vi "Session_from_previous_session_dialog.vi"(8 "Current Session Information":T4={"CollectionOfPoints"=[], "Instrument"=enum."Unknown", "CollectionFile"=path "kfaj;ldkfja;f", "Session Name/ID"="", "SessionNotes"=""}) -> (0 "Current Session Information Out":T4={"CollectionOfPoints"=[], "Instrument"=enum."Unknown", "CollectionFile"=path "kfaj;ldkfja;f", "Session Name/ID"="", "SessionNotes"=""}, 3 "Cancelled?":bool)   [LabVIEW 2011]
doc: "Use this template to create a dialog box. This template polls the state of the buttons on the front panel and does not use events. Use the Dialog Using Events template (not available in the Base package) to create a dialog box with event handling."
uses:
  cm2nm_sample_set.ctl
  cm2nm_coordinate_information_v2.ctl
  Instrument_type_enum_v2.ctl
  <vilib>/Analysis/Matrix/Datatypes/RealMatrix.ctl
  <vilib>/Analysis/Matrix/NI_Matrix.lvlib
panel:
  out "transformed with error":T1[](array[typedef])
  in  "Induce_error":dbl
  out "transformed":T1[](array[typedef])
  out "String":string
  out "B - vector offset":T2=[[-50940.89375198816], [16651.91756507725], [483.99442685727536]]
  out "A - Transformation Matrix":T2=[[774.391778229561, 631.2948989068436, 0.0], [-630.6602275509395, 772.5947325435925, 0.0], [2.0151348362659673, -7.982499934864615, 0.0]]
  out "Chosen Array":T1[](array[typedef])
  in  "Azimuth(deg)":dbl
  in  "Elevation (deg)":dbl
  in  "Scale":dbl
  in  "Z-off":dbl
  in  "Y-off":dbl
  in  "X-off":dbl
  in  "ChooseSpots":T3(array[cluster])
  in  "Cancel":bool
  in  "OK":bool
  # "Add the contents of your dialog here.\n\nTip: use controls from the System category of the Controls \npalette for professional appearance.\n\nReplace this text with your own, or delete this label."
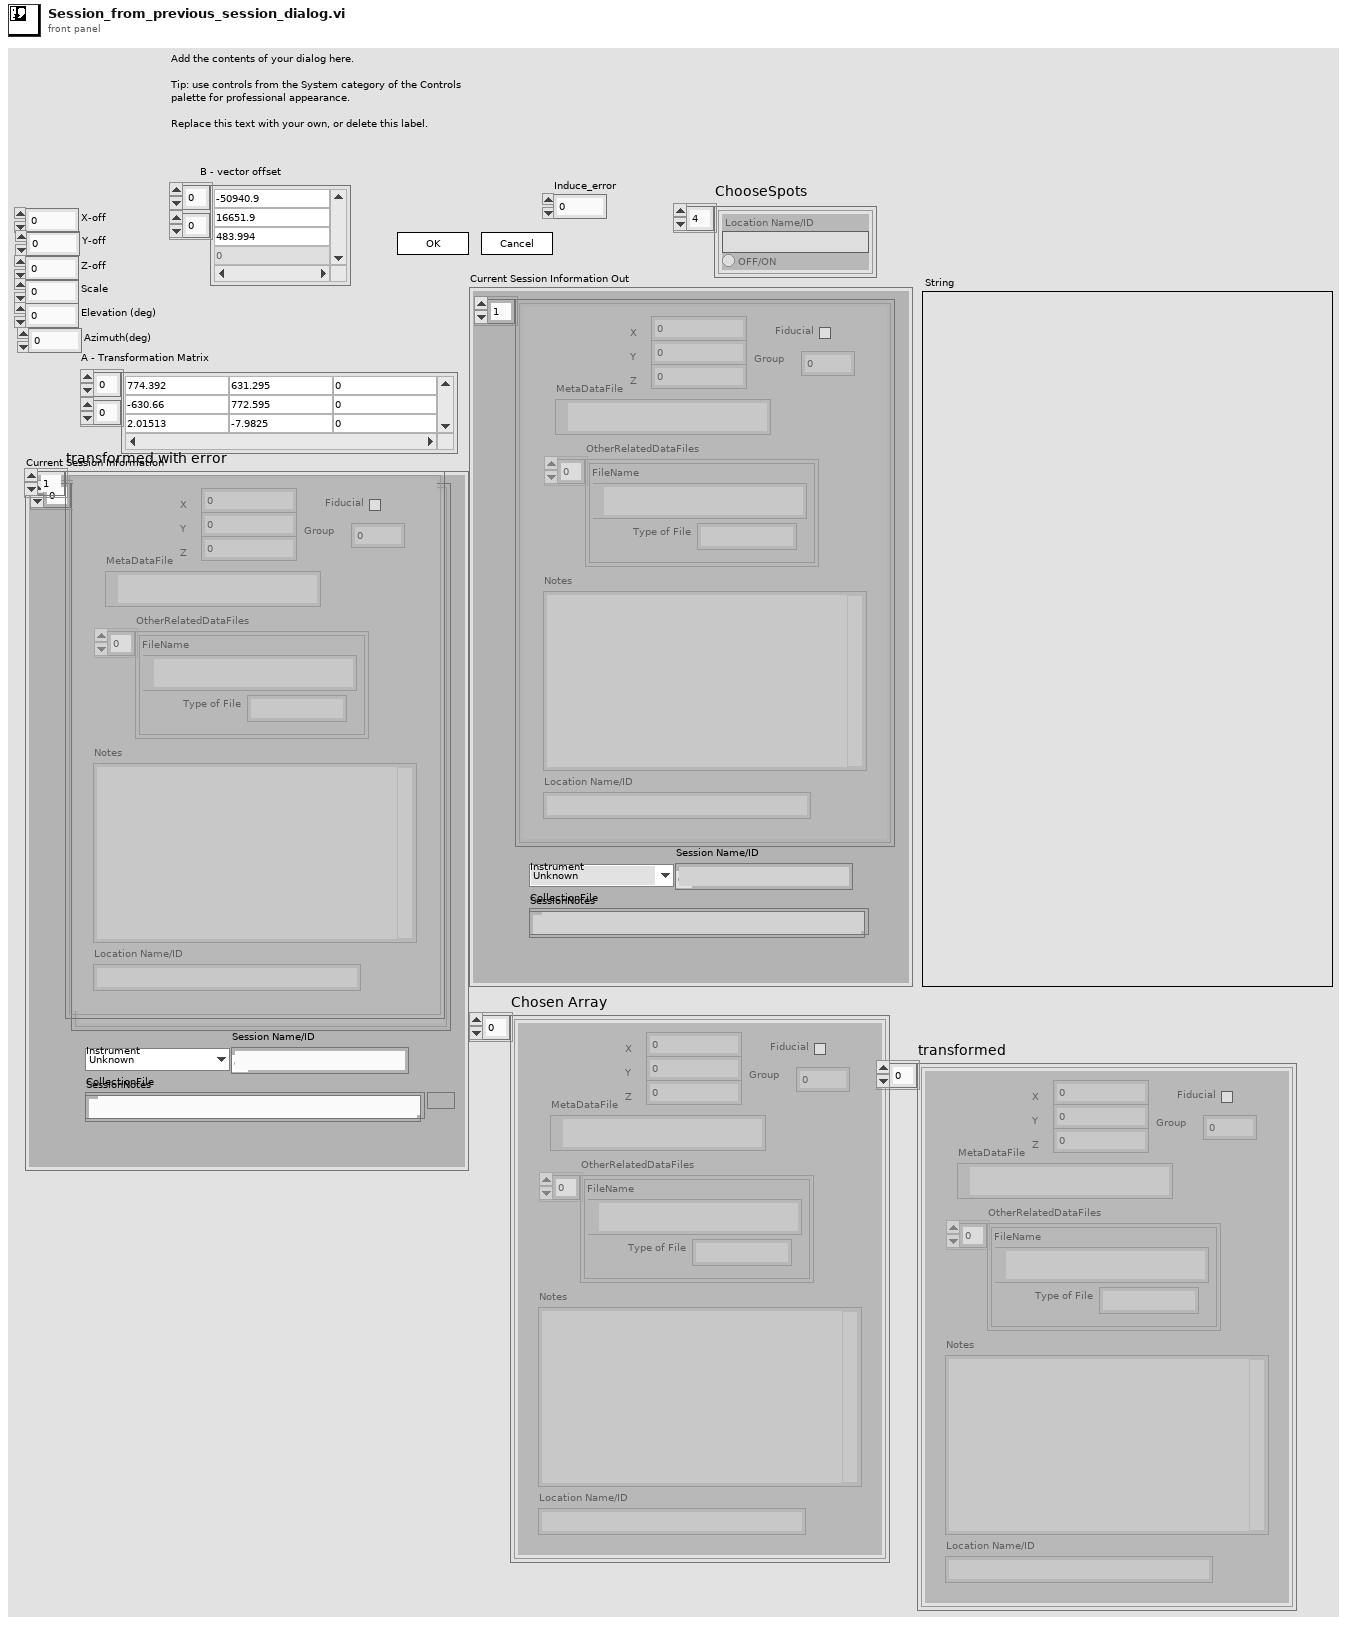
[diagram p1: front panel]
types:
  T1 = typedef "cm2nm_coordinate_information_v2.ctl" = cluster{"MetaDataFile":path, "X":dbl, "Y":dbl, "Z":dbl, "Group":i32, "Rotation":dbl[unit], "Fiducial":bool, "Magnification":dbl, "Working_Distance":dbl, "Notes":string, "Location Name/ID":string, "OtherRelatedDataFiles":cluster{"Type of File":string, "FileName":path}[], "Available":bool}
  T2 = typedef "NI_Matrix.lvlib/RealMatrix.ctl" = dbl[][]
  T3 = cluster{"Location Name/ID":string, "Choose":bool}[]
  T4 = typedef "cm2nm_sample_set.ctl" = cluster{"CollectionOfPoints":T1[], "Instrument":T5, "CollectionFile":path, "Session Name/ID":string, "SessionNotes":string}
  T5 = typedef "Instrument_type_enum_v2.ctl" = enum16{"Unknown", "Philips FEI SEM IRC", "JEOL 7000F EML_MFC", "MXRD MFC", "JEOL_EPMA"}
  T6 = cluster{"Location Name/ID":string, "select":bool}
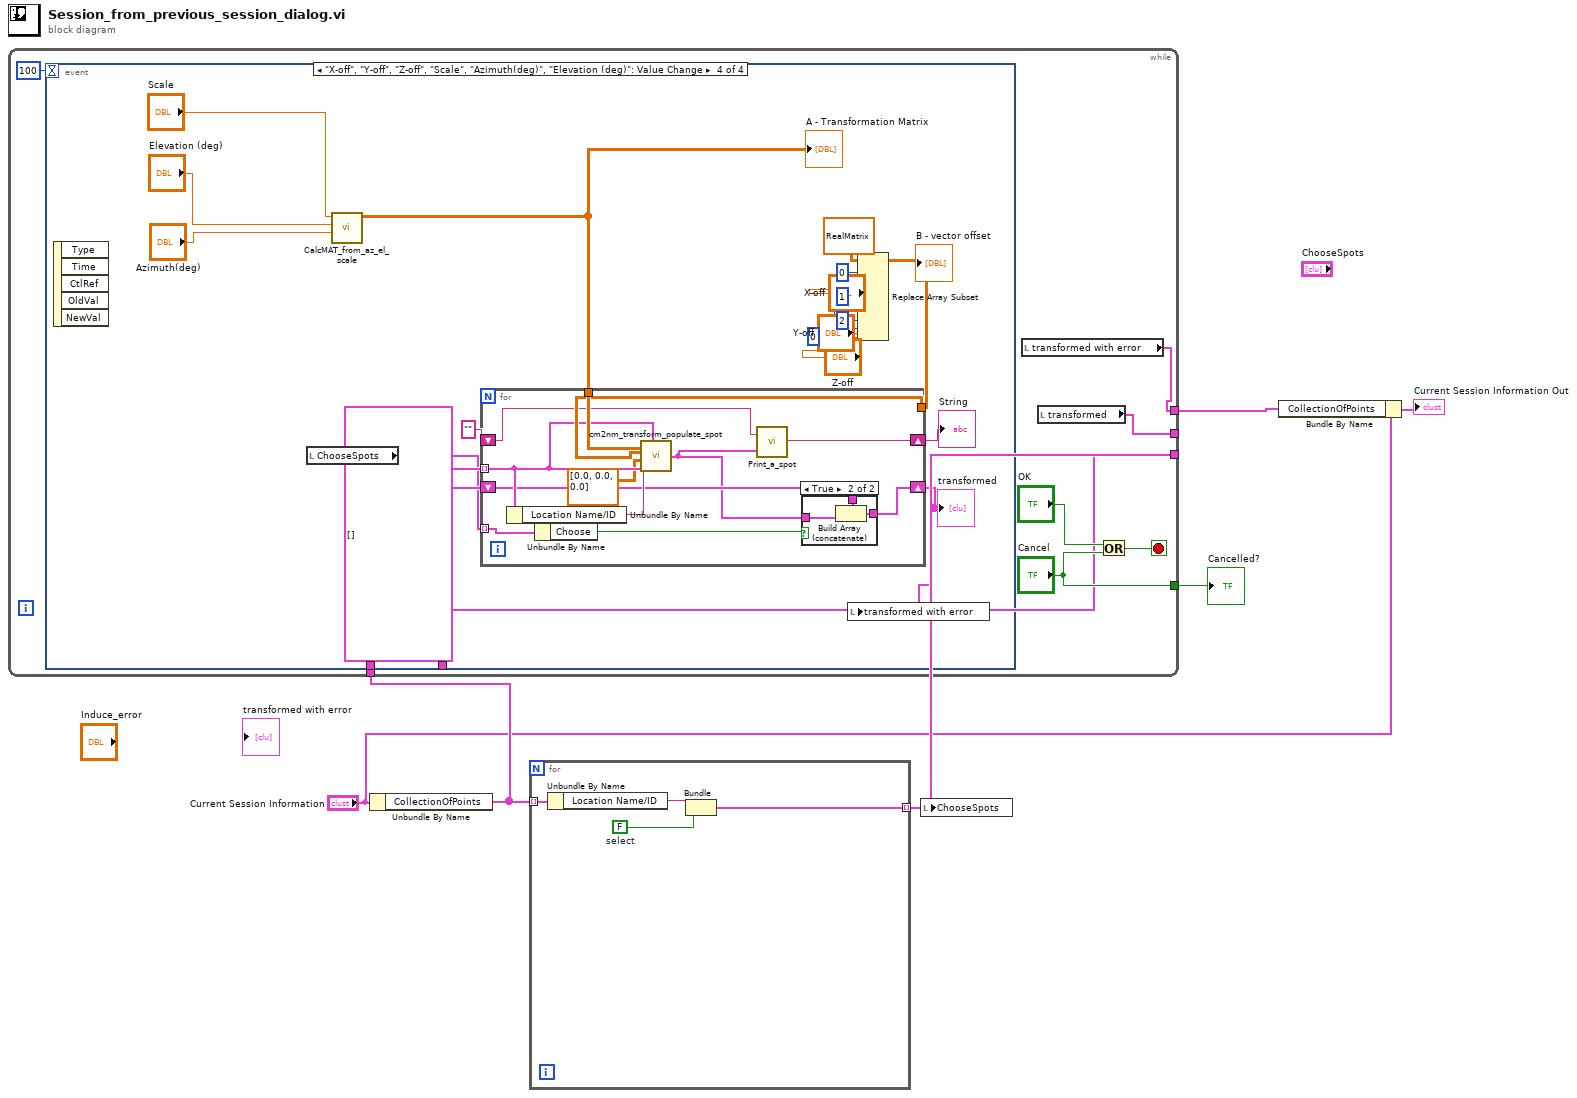
[diagram p0: block diagram]
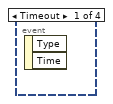
[diagram p2: hidden frame]
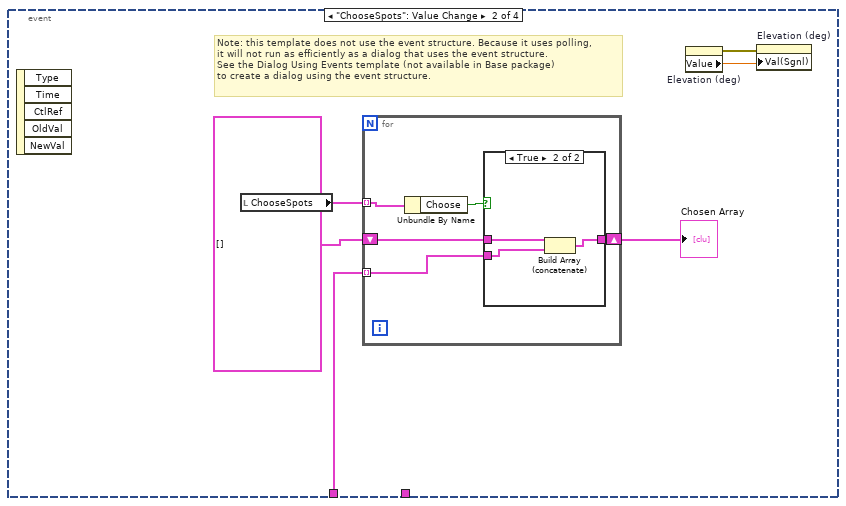
[diagram p3: hidden frame]
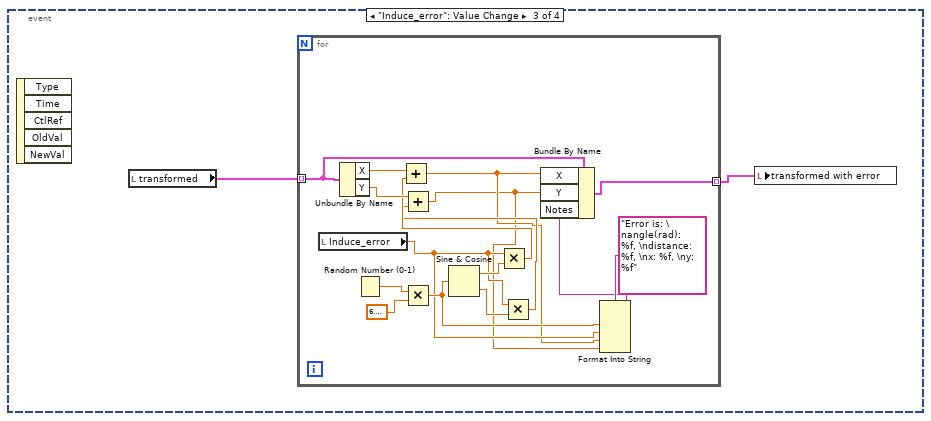
[diagram p5: hidden frame]
diagram:
  n1 = Unbundle By Name("Current Session Information") -> ("CollectionOfPoints"=w5:T1[])
  n2 = for {
    tunnel: w5 -> [w10] mode=indexing
    tunnel: [w7] -> w4 mode=indexing
    w8 = FALSE  # select
    n3 = Unbundle By Name(w10) -> ("Location Name/ID"=w9:string)
    n4 = Bundle("Location Name/ID"=w9, "select"=w8) -> (w7:T6)  [unwired: 1 in]
  }
  n5 = while {
    tunnel: ["Cancel"] -> w6
    tunnel: w5 -> [w15]
    tunnel: w4 -> [w13]
    tunnel: [w12] -> w1
    tunnel: [w11] -> _
    stop <- w17 stop-if-true
    n6 = event shown="[3] \"X-off\", \"Y-off\", \"Z-off\", \"Scale\", \"Azimuth(deg)\", \"Elevation (deg)\": Value Change" {
      selector: _ -> [_ _ _ _]
      dyn-events: _ -> [_ _ _ _]
      timeout: 100 -> [_ _ _ _]
      tunnel: w15 -> [_ w24 _ w54]
      tunnel: w13 -> [_ _ _ _]
      event Timeout {
        n7 = event-data() -> ()  [unwired: 1 in, 2 out]
      }
      event "ChooseSpots": Value Change {
        # "Note: this template does not use the event structure. Because it uses polling, \nit will not run as efficiently as a dialog that uses the event structure.\nSee the Dialog Using Events template (not available in Base package) \nto create a dialog using the event structure."
        n8 = event-data() -> ()  [unwired: 1 in, 5 out]
        n9 = local read "ChooseSpots"() -> (w23:T3)
        n10 = for {
          tunnel: w24 -> [w27] mode=indexing
          tunnel: w23 -> [w29] mode=indexing
          shift-right: [w25] -> w21
          shift-left: T1[] [] -> [w26]
          n11 = Unbundle By Name(w29) -> ("Choose"=w28:bool)
          n12 = case shown="True" w28 {
            tunnel: w27 -> [_ w32]
            tunnel: w26 -> [w30 w33]
            tunnel: [w30 w31] -> w25
            frame False {
            }
            frame True {
              n13 = Build Array (concatenate)(w33, w32) -> (w31:T1[])
            }
          }
        }
        "Chosen Array" <- w21
        n14 = property on="Elevation (deg)" class="DigNum (strict)"() -> (error out=w19:errorcluster, "Value"=w20:dbl)  [unwired: 2 in, 1 out]
        n15 = property on="Elevation (deg)" class="DigNum (strict)"(error in=w19, "Val(Sgnl)"=w20) -> ()  [unwired: 1 in, 2 out]
      }
      event "Induce_error": Value Change {
        n16 = event-data() -> ()  [unwired: 1 in, 5 out]
        n17 = local read "transformed"() -> (w35:T1[])
        n18 = for {
          tunnel: w35 -> [w51] mode=indexing
          tunnel: [w46] -> w34 mode=indexing
          n19 = local read "Induce_error"() -> (w39:dbl)
          n20 = Unbundle By Name(w51) -> ("X"=w45:dbl, "Y"=w44:dbl)
          n21 = Random Number (0-1)() -> (number: 0 to 1=w50:dbl)
          n22 = Multiply(x=w50, y=6.283185307179586) -> (x*y=w41:dbl)
          n23 = Sine & Cosine(0:w41) -> (1:w48:dbl, 2:w47:dbl)
          n24 = Multiply(x=w39, y=w48) -> (x*y=w43:dbl)
          n25 = Add(x=w45, y=w43) -> (x+y=w38:dbl)
          n26 = Multiply(x=w39, y=w47) -> (x*y=w42:dbl)
          n27 = Add(x=w44, y=w42) -> (x+y=w37:dbl)
          n28 = Format Into String(format string="Error is: \nangle(rad): %f, \ndistance: %f, \nx: %f, \ny: %f", w41, w39, w38, w37) -> (resulting string=w36:string)  [unwired: 2 in, 1 out]
          n29 = Bundle By Name(cluster=w51, "X"=w38, "Y"=w37, "Notes"=w36) -> (w46:T1)
        }
        n30 = local write "transformed with error"(w34) -> ()
      }
      event "X-off", "Y-off", "Z-off", "Scale", "Azimuth(deg)", "Elevation (deg)": Value Change {
        w67 = 0 ("disabled index (col)")
        n31 = event-data() -> ()  [unwired: 1 in, 5 out]
        n32 = local read "ChooseSpots"() -> (w53:T3)
        n33 = call "CalcMAT_from_az_el_scale.vi"("Azimuth(deg)"="Azimuth(deg)", "Elevation (deg)"="Elevation (deg)", "Scale"="Scale") -> ("A"=w58:T2)  [unwired: 8 in]
        "A - Transformation Matrix" <- w58
        n34 = Replace Array Subset(array=T2 [[-5.2614775143844385e-06], [-6.52811138479592e-15], [2.4868995751603505e-15]] ("B - vector offset"), new element #1="X-off", index (row) #1=0 ("index (row)"), index (col) #1=w67, new element #2="Y-off", index (row) #2=1 ("disabled index (row)"), index (col) #2=w67, new element #3="Z-off", index (row) #3=2 ("disabled index (row)"), index (col) #3=w67) -> (w62:T2)
        "B - vector offset" <- w62
        n35 = for {
          tunnel: w62 -> [w81]
          tunnel: w58 -> [w82]
          tunnel: w54 -> [w77] mode=indexing
          shift-right: [w80] -> w57
          shift-left: "" -> [w79]
          tunnel: w53 -> [w73] mode=indexing
          shift-right: [w74] -> w52
          shift-left: T1[] [] -> [w76]
          n36 = Unbundle By Name(w77) -> ("Location Name/ID"=w78:string)
          n37 = Unbundle By Name(w73) -> ("Choose"=w72:bool)
          n38 = call "cm2nm_transform_populate_spot.vi"("NewPointIn"=w77, "A - Transformation Matrix"=w82, "Previous Session Spot"=w77, "C"=T2 [[0.0], [0.0], [0.0]] ("B - vector offset"), "B - vector offset"=w81, "Spot_ID"=w78) -> ("NewPointOut"=w75:T1)
          n39 = call "Print_a_spot.vi"("Position"=w75, "String In"=w79) -> ("String Out"=w80:string)
          n40 = case shown="True" w72 {
            tunnel: w76 -> [w83 w86]
            tunnel: w75 -> [_ w85]
            tunnel: [w83 w84] -> w74
            frame False {
            }
            frame True {
              n41 = Build Array (concatenate)(w86, w85) -> (w84:T1[])
            }
          }
        }
        "String" <- w57
        "transformed" <- w52
        n42 = local write "transformed with error"(w52) -> ()
      }
    }
    n43 = local read "transformed with error"() -> (w12:T1[])
    n44 = local read "transformed"() -> (w11:T1[])
    n45 = Or(x="OK", y="Cancel") -> (x .or. y?=w17:bool)
  }
  "Cancelled?" <- w6
  n46 = local write "ChooseSpots"(w4) -> ()
  n47 = Bundle By Name(cluster="Current Session Information", "CollectionOfPoints"=w1) -> (→"Current Session Information Out":T4)
